vi "DMM DCVM Configure and Measure Only in a Loop.vi"() -> ()   [LabVIEW 2021]
uses:
  DMM_DC-RMS Voltage Measurement/Typedefs/Function Settings.ctl
  <instrlib>/niDMM/nidmm.llb/niDMM Resolution in Digits.ctl
  DMM_DC-RMS Voltage Measurement/Typedefs/Timing & Trigger Settings.ctl
  <instrlib>/niDMM/nidmm.llb/niDMM Trigger.ctl
  <instrlib>/niDMM/nidmm.llb/niDMM Slope.ctl
  DMM_DC-RMS Voltage Measurement/Typedefs/Measurement.ctl
  DMM Mixed Measurements/DMM Mixed Meas Typedefs/DMM Execution Settings.ctl
  <instrlib>/niDMM/nidmm.llb/niDMM Powerline Frequency.ctl
  Common/Typedefs/Execution Options - Measure.ctl
  DMM_DC-RMS Voltage Measurement/DMM_DC-RMS Voltage Measurement.lvlib
  DMM Mixed Measurements/DMM_Mixed Measurement.lvlib
panel:
  out "error out":errorcluster
  out "DMM Execution Settings":T1={"Absolute\nResolution"=0.0, "Input Resistance\n(Ohm)"=10000000.0, "Digits\nResolution"=5.5, "Range"=-1.0, "Minimum\nFrequency (Hz)"=20.0, "Aperture\nTime (s)"=0.0004999999999999999, "Auto Range\nValue"=10.0, "Settle\nTime (s)"=0.002, "Function"=1} {"Function" items=["DC Volts"=1, "AC Volts"=2, "DC Current"=3, "AC Current"=4, "2-Wire Resistance"=5, "4-Wire Resistance"=101, "Frequency"=104, "Period"=105, "AC Volts DC Coupled"=1001, "Diode"=1002, "Waveform Voltage"=1003, "Waveform Current"=1004, "Capacitance"=1005, "Inductance"=1006, "Temperature"=108]; "Absolute\nResolution" format="%#_6p"; "Input Resistance\n(Ohm)" format="%#_6p"; "Range" format="%#_6p"; "Minimum\nFrequency (Hz)" format="%#_6p"; "Aperture\nTime (s)" format="%#_6p"; "Auto Range\nValue" format="%#_6p"; "Settle\nTime (s)" format="%#_6p"}
  out "Measurement":T2={"Measured Value"=9.996587808477924, "Out of Range"=FALSE, "Unit"="V (dc)", "Measurement"="9.99659V (dc)"} {"Measured Value" format="%^#_9e"}
  in  "Stop Button":bool
  in  "Timing and Trigger Settings":T3={"AC Min Frequency (Hz)"=40.0, "Aperture Time (s)"=-1.0, "Settle Time (s)"=-1.0, "Trigger Settings"={"Trigger Delay (sec)"=-1.0, "Enable Trigger?"=FALSE, "Trigger Source"=enum."Immediate", "Slope"=enum."Rising Edge"}} {"Trigger Settings"."Trigger Delay (sec)" format="%.4f"; "AC Min Frequency (Hz)" format="%.2f"}
  in  "Function Settings":T6={"Range and Function"=enum."DC Voltage Auto Range", "Resolution in Digits"=5.5} {"Resolution in Digits" items=["3 1/2"=3.5, "4 1/2"=4.5, "5 1/2"=5.5, "6 1/2"=6.5, "7 1/2"=7.5]}
  in  "DMM Resource Name":refnum<k15>="DMM_4080"
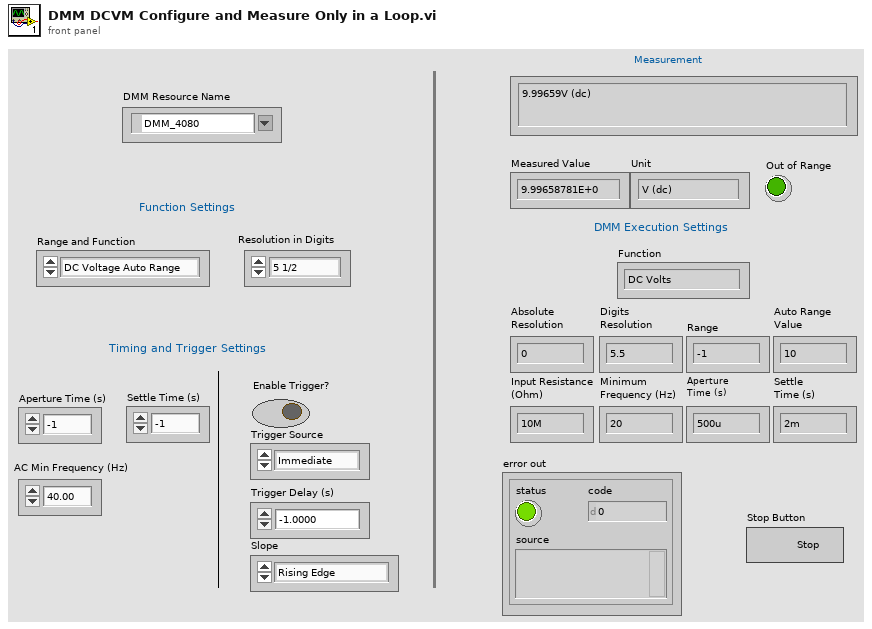
[diagram p1: front panel]
types:
  T1 = typedef "DMM_Mixed Measurement.lvlib/DMM Execution Settings.ctl" = cluster{"Absolute\nResolution":dbl, "Input Resistance\n(Ohm)":dbl, "Digits\nResolution":dbl, "Range":dbl, "Minimum\nFrequency (Hz)":dbl, "Aperture\nTime (s)":dbl, "Auto Range\nValue":dbl, "Settle\nTime (s)":dbl, "Function":i32}
  T2 = typedef "DMM_DC-RMS Voltage Measurement.lvlib/Measurement.ctl" = cluster{"Measured Value":dbl, "Out of Range":bool, "Unit":string, "Measurement":string}
  T3 = typedef "DMM_DC-RMS Voltage Measurement.lvlib/Timing & Trigger Settings.ctl" = cluster{"AC Min Frequency (Hz)":dbl, "Aperture Time (s)":dbl, "Settle Time (s)":dbl, "Trigger Settings":cluster{"Trigger Delay (sec)":dbl, "Enable Trigger?":bool, "Trigger Source":T4, "Slope":T5}}
  T4 = typedef "niDMM Trigger.ctl" = enum16{"Immediate", "External", "TTL 0", "TTL 1", "TTL 2", "TTL 3", "TTL 4", "TTL 5", "TTL 6", "Software", "TTL 7", "PXI Star", "LBR Trig 1", "Aux Trig 1"}
  T5 = typedef "niDMM Slope.ctl" = enum16{"Rising Edge", "Falling Edge"}
  T6 = typedef "DMM_DC-RMS Voltage Measurement.lvlib/Function Settings.ctl" = cluster{"Range and Function":enum16{"DC Voltage Auto Range", "DC 100 mV", "DC 1 V ", "DC 10 V", "DC 100 V", "DC 300 V", " ", "AC Voltage Auto Range", "AC 50 mV", "AC 200 mV", "AC 500 mV", "AC 2 V", "AC 5 V", "AC 20 V", "AC 50 V", "AC 300 V"}, "Resolution in Digits":T7}
  T7 = typedef "niDMM Resolution in Digits.ctl" = dbl
  T8 = typedef "Execution Options - Measure.ctl" = enum16{"Configure & Measure", "Configure only", "Measure only"}
  T9 = typedef "niDMM Powerline Frequency.ctl" = enum16{"60 Hz", "50 Hz"}
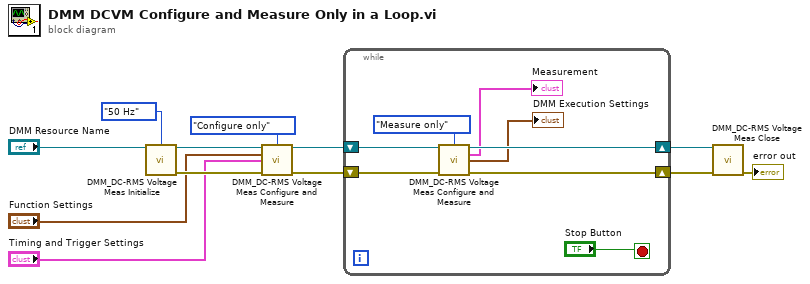
[diagram p0: block diagram]
diagram:
  n1 = call "DMM_DC-RMS Voltage Meas Initialize.vi"("DMM Resource Name"="DMM Resource Name", "Powerline Frequency"=niDMM_Powerline_Frequency."50 Hz") -> ("DMM Handle Out"=w12:refnum<k15>, "error out"=w11:errorcluster)  [unwired: 12 in]
  n2 = call "DMM_DC-RMS Voltage Meas Configure and Measure.vi"("DMM Handle In"=w12, "Execution Option"=Execution_Options_-_Measure."Configure only", "Function Settings"="Function Settings", "Timing and Trigger Settings"="Timing and Trigger Settings", "error in"=w11) -> ("DMM Handle Out"=w10:refnum<k15>, "error out"=w9:errorcluster)  [unwired: 7 in, 2 out]
  n3 = while {
    shift-right: [w18] -> w8
    shift-left: w10 -> [w20]
    shift-right: [w17] -> w7
    shift-left: w9 -> [w19]
    stop <- "Stop Button" stop-if-true
    n4 = call "DMM_DC-RMS Voltage Meas Configure and Measure.vi"("DMM Handle In"=w20, "Execution Option"=Execution_Options_-_Measure."Measure only", "error in"=w19) -> ("DMM Handle Out"=w18:refnum<k15>, "Measurement"=→"Measurement":T2, "DMM Execution Settings"=→"DMM Execution Settings":T1, "error out"=w17:errorcluster)  [unwired: 9 in]
  }
  n5 = call "DMM_DC-RMS Voltage Meas Close.vi"("DMM Handle In"=w8, "error in"=w7) -> ("error out"=→"error out":errorcluster)  [unwired: 13 in]
